vi "1.vi"() -> ()   [LabVIEW 2022 SP3]
uses:
  LABVIEW FILE'S/comman 2.o.vi
panel:
  in  "stop":bool
  in  "Seek Forward Button":bool
  out "output array":string[](array[string])
  in  "Enum":T1(ring)
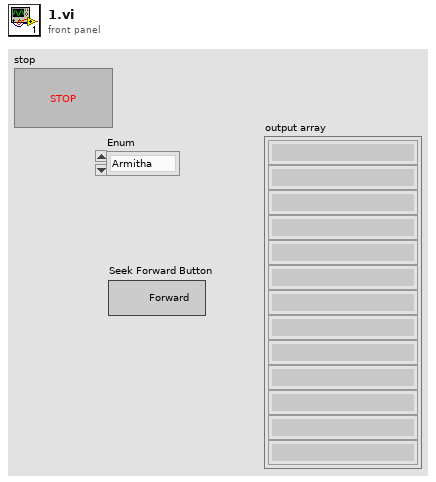
[diagram p1: front panel]
types:
  T1 = enum16{"Armitha", "Janani", "Thara", "Shaikthi", "Pairvatha", ""}
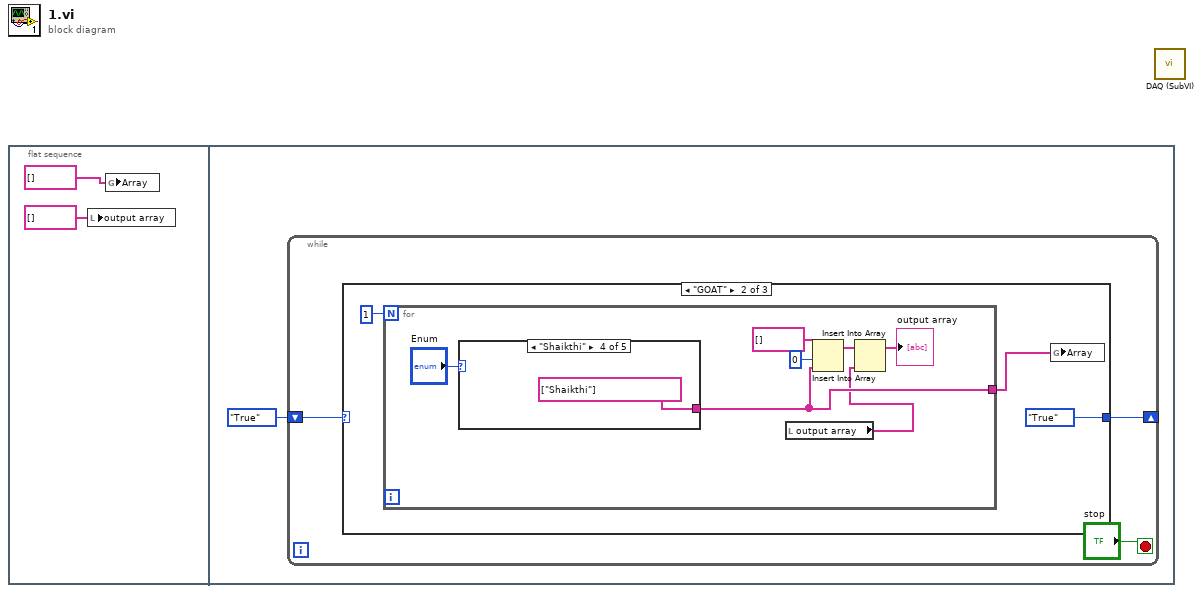
[diagram p0: block diagram]
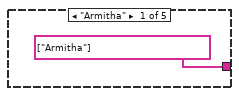
[diagram p3: hidden frame]
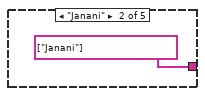
[diagram p4: hidden frame]
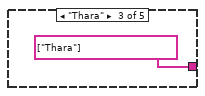
[diagram p5: hidden frame]
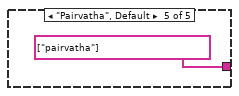
[diagram p6: hidden frame]
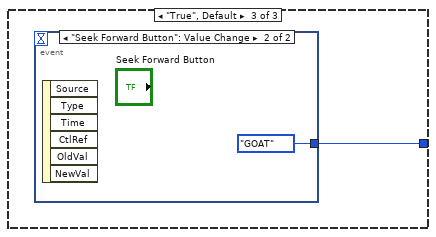
[diagram p7: hidden frame]
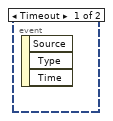
[diagram p8: hidden frame]
diagram:
  n1 = flat-sequence {
    frame #0 {
      n2 = local write "output array"(string[] [] ("output array")) -> ()
      n3 = global write "comman 2.o.vi" "Array"(string[] []) -> ()
    }
    frame #1 {
      n4 = while {
        shift-right: [w5] -> _
        shift-left: enum16{"False", "True", "GOAT"}."True" -> [w6]
        stop <- "stop" stop-if-true
        n5 = case shown="\"GOAT\"" w6 {
          tunnel: [_ enum16{"False", "True", "GOAT"}."True" w22] -> w5
          frame "False" {
          }
          frame "GOAT" {
            n6 = for {
              N: 1 -> [_]
              tunnel: [w14] -> w7
              n7 = case shown="\"Shaikthi\"" "Enum" {
                tunnel: [string[] ["Armitha"] string[] ["Janani"] string[] ["Thara"] string[] ["Shaikthi"] string[] ["pairvatha"]] -> w14
                frame "Armitha" {
                }
                frame "Janani" {
                }
                frame "Thara" {
                }
                frame "Shaikthi" {
                }
                frame "Pairvatha", Default {
                }
              }
              n8 = local read "output array"() -> (w11:string[])
              n9 = Insert Into Array(array=string[] [], index=0, new element=w14) -> (w13:string[])
              n10 = Insert Into Array(array=w13, new element=w11) -> (→"output array":string[])  [unwired: 1 in]
            }
            n11 = global write "comman 2.o.vi" "Array"(w7) -> ()
          }
          frame "True", Default {
            n12 = event shown="[1] \"Seek Forward Button\": Value Change" {
              selector: _ -> [_ _]
              dyn-events: _ -> [_ _]
              timeout: _ -> [_ _]
              tunnel: [_ enum16{"False", "True", "GOAT"}."GOAT"] -> w22
              event Timeout {
                n13 = event-data() -> ()  [unwired: 1 in, 3 out]
              }
              event "Seek Forward Button": Value Change {
                n14 = event-data() -> ()  [unwired: 1 in, 6 out]
              }
            }
          }
        }
      }
    }
  }
  n15 = call "DAQ (SubVI).vi"() -> ()  [unwired: 12 in]
